vi "StartPhidget.vi"   [LabVIEW 2012]
uses:
  <instrlib>/Phidgets/Phidget Accelerometer/Phidget Accelerometer.lvlib
  <instrlib>/Phidgets/Phidget Current Input/Phidget Current Input.lvlib
  <instrlib>/Phidgets/Phidget DC Motor/Phidget DC Motor.lvlib
  <instrlib>/Phidgets/Phidget Digital Input/Phidget Digital Input.lvlib
  <instrlib>/Phidgets/Phidget Digital Output/Phidget Digital Output.lvlib
  <instrlib>/Phidgets/Phidget Encoder/Phidget Encoder.lvlib
  <instrlib>/Phidgets/Phidget Frequency Counter/Phidget Frequency Counter.lvlib
  <instrlib>/Phidgets/Phidget GPS/Phidget GPS.lvlib
  <instrlib>/Phidgets/Phidget Gyroscope/Phidget Gyroscope.lvlib
  <instrlib>/Phidgets/Phidget Humidity Sensor/Phidget Humidity Sensor.lvlib
  <instrlib>/Phidgets/Phidget IR/Phidget IR.lvlib
  <instrlib>/Phidgets/Phidget LCD/Phidget LCD.lvlib
  <instrlib>/Phidgets/Phidget Light Sensor/Phidget Light Sensor.lvlib
  <instrlib>/Phidgets/Phidget Magnetometer/Phidget Magnetometer.lvlib
  <instrlib>/Phidgets/Phidget Pressure Sensor/Phidget Pressure Sensor.lvlib
  <instrlib>/Phidgets/Phidget RC Servo/Phidget RC Servo.lvlib
  <instrlib>/Phidgets/Phidget RFID/Phidget RFID.lvlib
  <instrlib>/Phidgets/Phidget Spatial/Phidget Spatial.lvlib
  <instrlib>/Phidgets/Phidget Stepper/Phidget Stepper.lvlib
  <instrlib>/Phidgets/Phidget Temperature Sensor/Phidget Temperature Sensor.lvlib
  <instrlib>/Phidgets/Phidget Voltage Input/Phidget Voltage Input.lvlib
  <instrlib>/Phidgets/Phidget Voltage Output/Phidget Voltage Output.lvlib
  <instrlib>/Phidgets/Phidget Voltage Ratio Input/Phidget Voltage Ratio Input.lvlib
  <instrlib>/Phidgets/Phidget Capacitive Touch/Phidget Capacitive Touch.lvlib
  <instrlib>/Phidgets/Phidget PH Sensor/Phidget PH Sensor.lvlib
  <instrlib>/Phidgets/Phidget Distance Sensor/Phidget Distance Sensor.lvlib
  <instrlib>/Phidgets/Phidget Sound Sensor/Phidget Sound Sensor.lvlib
  <instrlib>/Phidgets/Phidget Resistance Input/Phidget Resistance Input.lvlib
  <instrlib>/Phidgets/Phidget Power Guard/Phidget Power Guard.lvlib
  <instrlib>/Phidgets/Phidget Motor Position Controller/Phidget Motor Position Controller.lvlib
  <instrlib>/Phidgets/Phidget BLDC Motor/Phidget BLDC Motor.lvlib
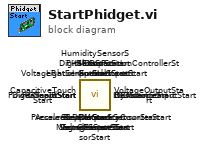
[diagram p0: block diagram]
diagram:
  n1 = call <instrlib>:"BLDCMotorStart.vi"() -> ()  [unwired: 12 in, 4 out]
  n2 = call <instrlib>:"MotorPositionControllerStart.vi"() -> ()  [unwired: 12 in, 4 out]
  n3 = call <instrlib>:"PowerGuardStart.vi"() -> ()  [unwired: 12 in, 4 out]
  n4 = call <instrlib>:"ResistanceInputStart.vi"() -> ()  [unwired: 12 in, 4 out]
  n5 = call <instrlib>:"SoundSensorStart.vi"() -> ()  [unwired: 12 in, 4 out]
  n6 = call <instrlib>:"VoltageRatioInputStart.vi"() -> ()  [unwired: 12 in, 4 out]
  n7 = call <instrlib>:"DistanceSensorStart.vi"() -> ()  [unwired: 12 in, 4 out]
  n8 = call <instrlib>:"PHSensorStart.vi"() -> ()  [unwired: 12 in, 4 out]
  n9 = call <instrlib>:"CapacitiveTouchStart.vi"() -> ()  [unwired: 12 in, 4 out]
  n10 = call <instrlib>:"VoltageOutputStart.vi"() -> ()  [unwired: 12 in, 4 out]
  n11 = call <instrlib>:"TemperatureSensorStart.vi"() -> ()  [unwired: 12 in, 4 out]
  n12 = call <instrlib>:"StepperStart.vi"() -> ()  [unwired: 12 in, 4 out]
  n13 = call <instrlib>:"SpatialStart.vi"() -> ()  [unwired: 12 in, 4 out]
  n14 = call <instrlib>:"RFIDStart.vi"() -> ()  [unwired: 12 in, 4 out]
  n15 = call <instrlib>:"RCServoStart.vi"() -> ()  [unwired: 12 in, 4 out]
  n16 = call <instrlib>:"PressureSensorStart.vi"() -> ()  [unwired: 12 in, 4 out]
  n17 = call <instrlib>:"MagnetometerStart.vi"() -> ()  [unwired: 12 in, 4 out]
  n18 = call <instrlib>:"LightSensorStart.vi"() -> ()  [unwired: 12 in, 4 out]
  n19 = call <instrlib>:"LCDStart.vi"() -> ()  [unwired: 12 in, 4 out]
  n20 = call <instrlib>:"IRStart.vi"() -> ()  [unwired: 12 in, 4 out]
  n21 = call <instrlib>:"HumiditySensorStart.vi"() -> ()  [unwired: 12 in, 4 out]
  n22 = call <instrlib>:"GyroscopeStart.vi"() -> ()  [unwired: 12 in, 4 out]
  n23 = call <instrlib>:"GPSStart.vi"() -> ()  [unwired: 12 in, 4 out]
  n24 = call <instrlib>:"FrequencyCounterStart.vi"() -> ()  [unwired: 12 in, 4 out]
  n25 = call <instrlib>:"EncoderStart.vi"() -> ()  [unwired: 12 in, 4 out]
  n26 = call <instrlib>:"DigitalOutputStart.vi"() -> ()  [unwired: 12 in, 4 out]
  n27 = call <instrlib>:"DigitalInputStart.vi"() -> ()  [unwired: 12 in, 4 out]
  n28 = call <instrlib>:"DCMotorStart.vi"() -> ()  [unwired: 12 in, 4 out]
  n29 = call <instrlib>:"CurrentInputStart.vi"() -> ()  [unwired: 12 in, 4 out]
  n30 = call <instrlib>:"AccelerometerStart.vi"() -> ()  [unwired: 12 in, 4 out]
  n31 = call <instrlib>:"VoltageInputStart.vi"() -> ()  [unwired: 12 in, 4 out]
